vi "SVG2EMF_JAR.vi"(6 "JAVA路径":path=path "C:/Program Files/Java/jre7/bin/javaw.exe", 8 "Error in":errorcluster caption="Error in (no error)", 10 "EMF路径":path, 11 "SVG":path) -> (0 "Error out":errorcluster)   [LabVIEW 2017]
uses:
  <userlib>/_OpenG.lib/file/file.llb/Convert File Extension (Path)__ogtk.vi
panel:
  out "standard error":string caption="标准错误"
  out "standard output":string caption="标准输出"
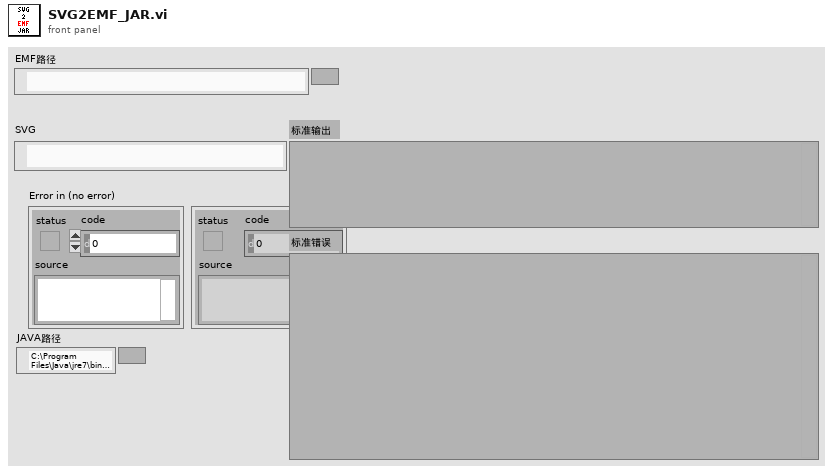
[diagram p1: front panel]
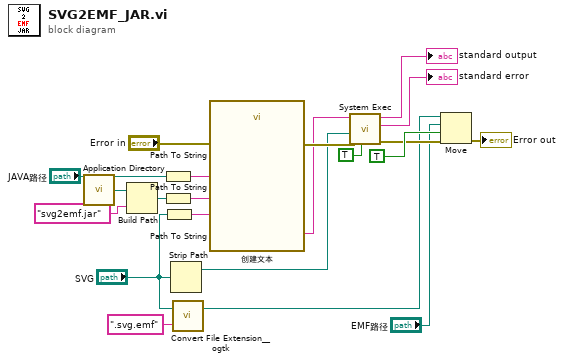
[diagram p0: block diagram]
diagram:
  n1 = call <vilib>:"Application Directory.vi"() -> ("Application Directory"=w16:path)
  n2 = Build Path(base path=w16, name or relative path="svg2emf.jar") -> (appended path=w3:path)
  n3 = Path To String(path="JAVA路径") -> (string=w2:string)
  n4 = Path To String(path=w3) -> (string=w4:string)
  n5 = Path To String(path="SVG") -> (string=w5:string)
  n6 = Strip Path(path="SVG") -> (stripped path=w11:path)  [unwired: 1 out]
  n7 = call-poly <userlib>:"Convert File Extension__ogtk.vi"("new ending (none)"=".svg.emf", "file name"="SVG") -> ("new filename"=w7:path)  [unwired: 1 out]
  n8 = call "创建文本"("java"=w2, "svg2emf.jar"=w4, "svg"=w5, "error in (no error)"="Error in") -> ("Result"=w12:string, "error out"=w13:errorcluster)  [unwired: 10 in]
  n9 = call <vilib>:"System Exec.vi"("run minimized? (F)"=TRUE, "error in (no error)"=w13, "working directory"=w11, "command line"=w12) -> ("error out"=w8:errorcluster, "standard error"=→"standard error":string, "standard output"=→"standard output":string)  [unwired: 4 in, 1 out]
  n10 = Move(source path=w7, error in=w8, 9:TRUE ("overwrite (F)"), 10:"EMF路径") -> (error out=→"Error out":errorcluster)  [unwired: 1 in, 2 out]
